vi "Excel_Write.vi"(4 "Cell Range 2":string="B1", 5 "Array To Write":dbl[][](array[numeric])=[[0.0]] format="%.6g", 6 "Cell Range 1":string="A1", 7 "Worksheet Number":i32=1, 8 "error in (no error)":errorcluster, 9 "Sheets Rerefence In":refnum<k7>) -> (0 "error out":errorcluster, 1 "Sheets Reference Out":refnum<k7>)   [LabVIEW 2014]
doc: "This VI demonstrates the use of ActiveX to write a table into a Microsoft Excel worksheet."
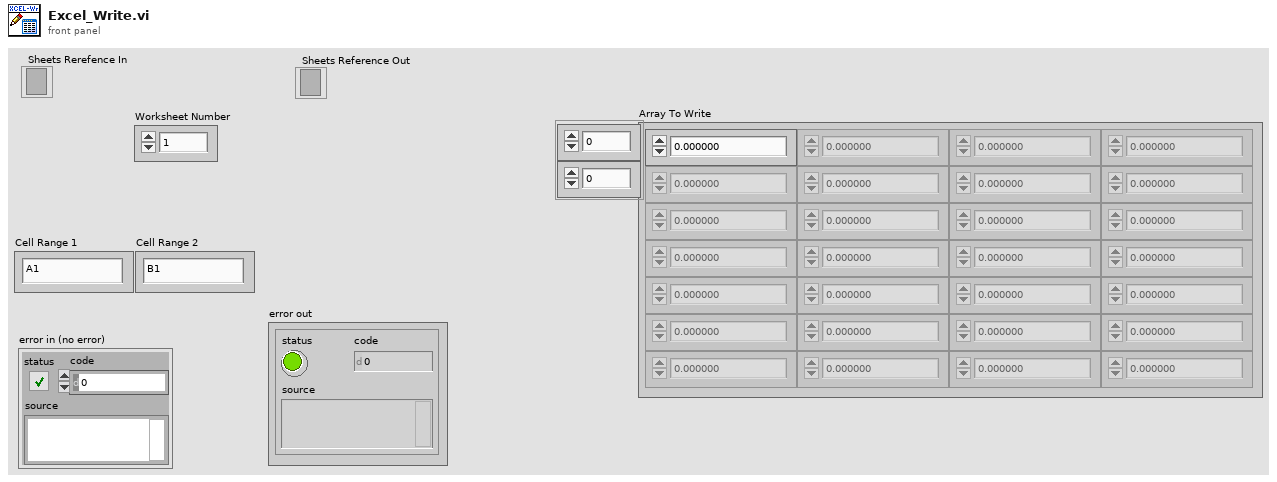
[diagram p1: front panel]
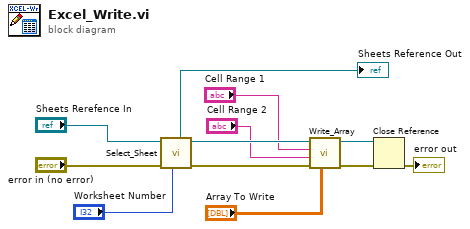
[diagram p0: block diagram]
diagram:
  n1 = call "Select_Sheet.vi"("Worksheet Number"="Worksheet Number", "error in (no error)"="error in (no error)", "Automation Refnum in"="Sheets Rerefence In") -> ("error out"=w12:errorcluster, "Automation Refnum out"=w11:refnum<k7>, "Sheets Refnum"=→"Sheets Reference Out":refnum<k7>)  [unwired: 6 in]
  n2 = call "Write_Array.vi"("Array To Write"="Array To Write", "error in (no error)"=w12, "Cell Range 2"="Cell Range 2", "Cell Range 1"="Cell Range 1", "Automation Refnum in"=w11) -> ("error out"=w3:errorcluster, "Automation Refnum out"=w4:refnum<k7>)  [unwired: 5 in]
  n3 = Close Reference(reference=w4, error in (no error)=w3) -> (error out=→"error out":errorcluster)
